vi "InitFromXML.vi"(8 "error in (no error)":errorcluster, 10 "XML":string, 11 "Link in":refnum<class "Link.lvclass">) -> (0 "error out":errorcluster, 3 "Link out":refnum<class "Link.lvclass">)   [LabVIEW 2009, in "NavScreen.lvlib" / "Link.lvclass"]
uses:
  Link.lvclass
  Link.lvclass/Link.ctl
  NavScreen.lvlib
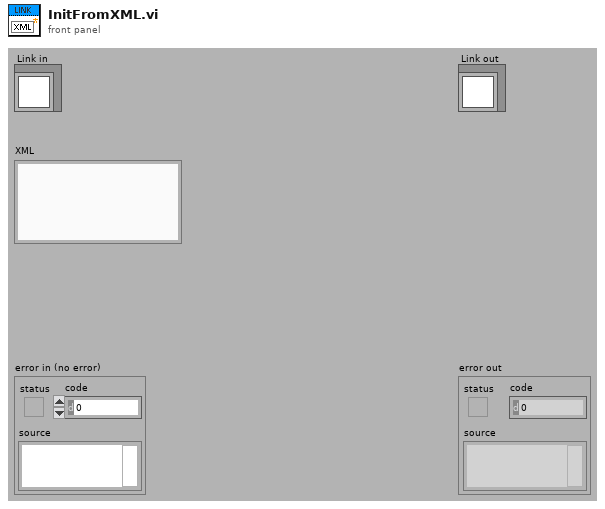
[diagram p1: front panel]
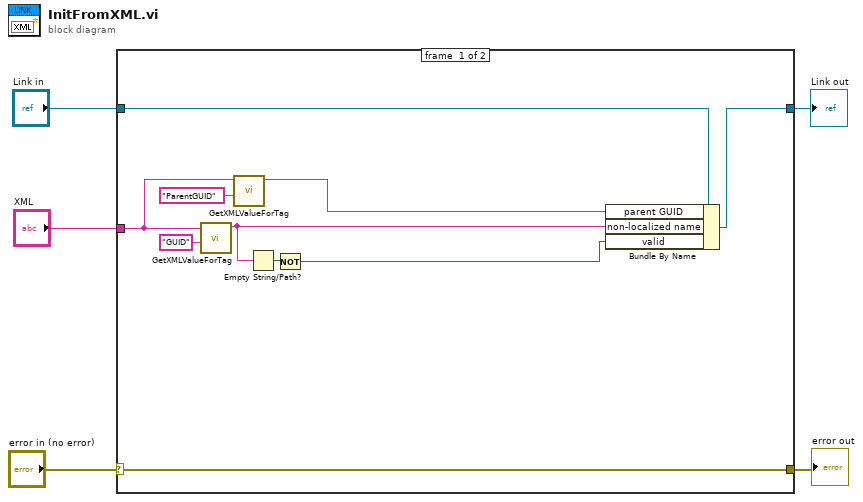
[diagram p0: block diagram]
diagram:
  n1 = case shown="No Error" "error in (no error)" {
    selector: "error in (no error)" -> [w15 w17]
    tunnel: [w15 w17] -> w4
    tunnel: [w13 w16] -> w2
    tunnel: "Link in" -> [w14 w16]
    tunnel: "XML" -> [w7 _]
    frame #0 {
      n2 = call "GetXMLValueForTag.vi"("tag"="GUID", "XML"=w7) -> ("value"=w12:string)  [unwired: 8 in, 1 out]
      n3 = call "GetXMLValueForTag.vi"("tag"="ParentGUID", "XML"=w7) -> ("value"=w8:string)  [unwired: 8 in, 1 out]
      n4 = Empty String/Path?(string/path=w12) -> (empty?=w11:bool)
      n5 = Not(x=w11) -> (.not. x?=w6:bool)
      n6 = Bundle By Name(cluster=w14, "parent GUID"=w8, "non-localized name"=w12, "valid"=w6) -> (w13:refnum<class "Link.lvclass">)
    }
    frame #1 {
    }
  }
  "error out" <- w4
  "Link out" <- w2
